vi "11_LAYOUT_COVID_19_BOTÓN.vi"() -> ()   [LabVIEW 2019]
panel:
  in  "vi path":path
  out "Numeric":i32
  in  "INT_TAB":bool
  in  "Tab Control":enum32{"Page 1", "Page 2"}(tab)
  out "Boolean":bool
  out "Boolean 2":bool
  in  "stop":bool
  # "LAYOUT --> TAB/SUB"
  # "SELECTOR TAB"
  # "(C) 2020"
  # "J.LUIS PÉREZ DEL VAL"
  # "GIF ANIMADO"
  # "KIT o CALENDARIO?..."
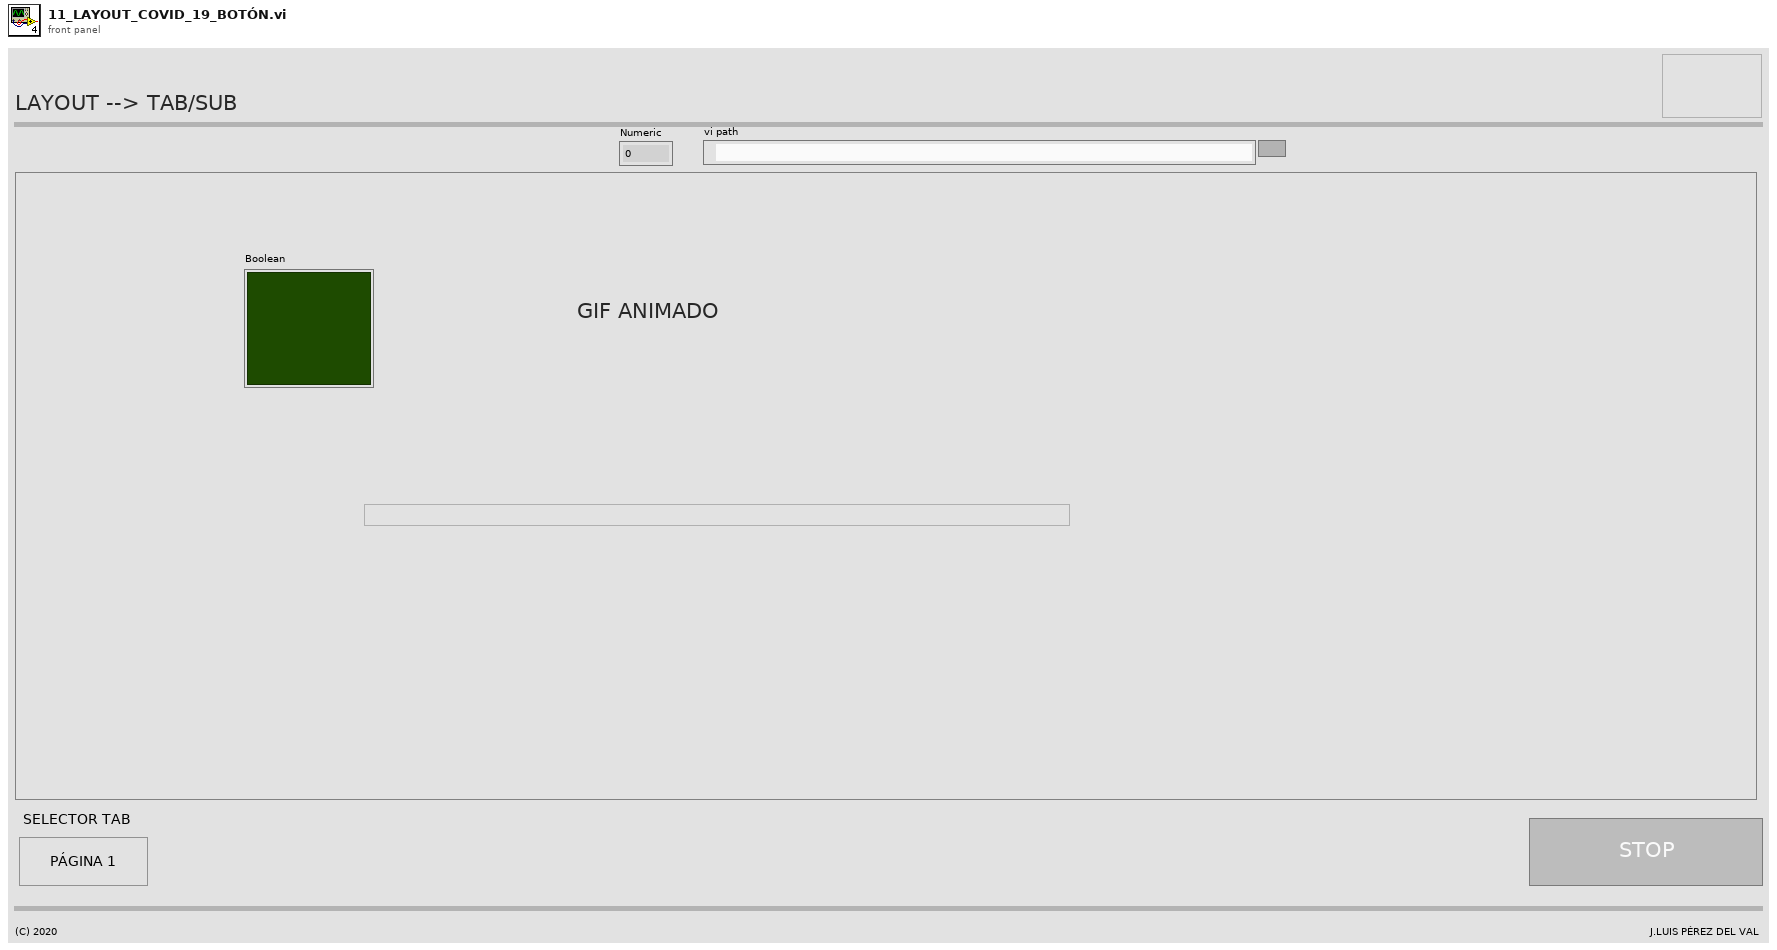
[diagram p1: front panel]
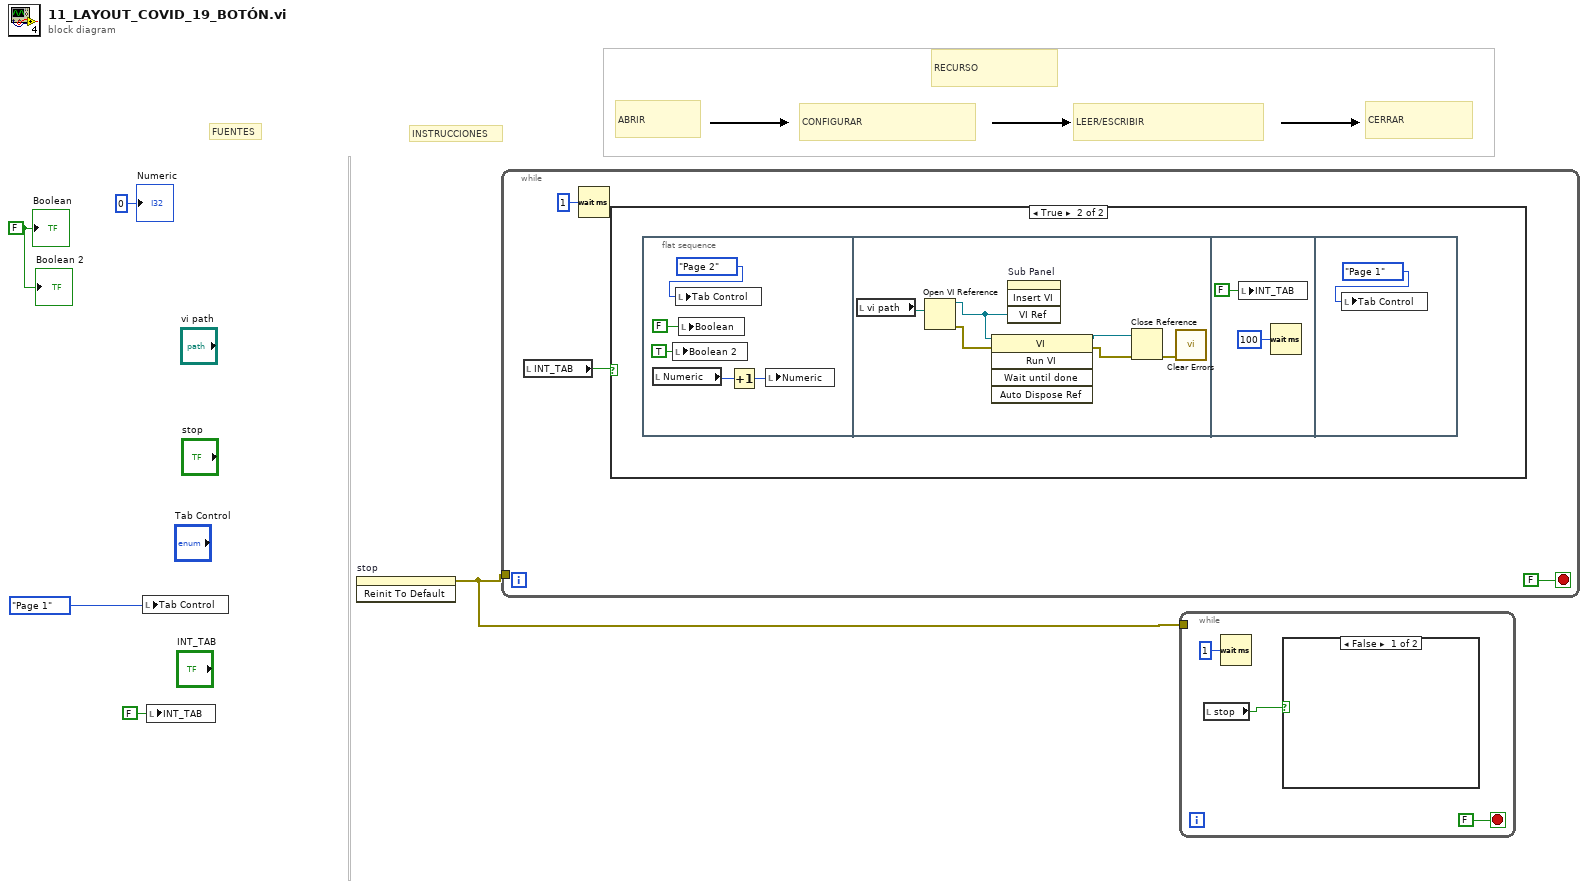
[diagram p0: block diagram]
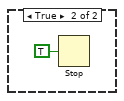
[diagram p2: hidden frame]
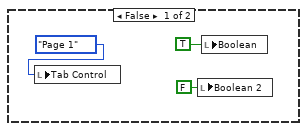
[diagram p3: hidden frame]
diagram:
  w2 = FALSE ("Boolean")
  # "RECURSO"
  # "CERRAR"
  # "LEER/ESCRIBIR"
  # "CONFIGURAR"
  # "ABRIR"
  # "INSTRUCCIONES"
  # "FUENTES"
  n1 = local write "Tab Control"(enum32{"Page 1", "Page 2"}."Page 1" ("Tab Control 2")) -> ()
  n2 = local write "INT_TAB"(FALSE ("INT_TAB")) -> ()
  n3 = invoke on="stop" class="Bool (strict)" method="Reinit To Default"() -> (error out=w5:errorcluster)  [unwired: 3 in, 2 out]
  n4 = while {
    tunnel: w5 -> [_]
    stop <- FALSE stop-if-true
    n5 = local read "INT_TAB"() -> (w6:bool)
    n6 = Wait (ms)(milliseconds to wait=u32 1) -> ()  [unwired: 1 out]
    n7 = case shown="True" w6 {
      frame False {
        n8 = local write "Tab Control"(enum32{"Page 1", "Page 2"}."Page 1" ("Tab Control 2")) -> ()
        n9 = local write "Boolean 2"(FALSE ("INT_TAB")) -> ()
        n10 = local write "Boolean"(TRUE ("INT_TAB")) -> ()
      }
      frame True {
        n11 = flat-sequence {
          frame #0 {
            n12 = local read "Numeric"() -> (w14:i32)
            n13 = local write "Boolean 2"(TRUE ("INT_TAB")) -> ()
            n14 = local write "Tab Control"(enum32{"Page 1", "Page 2"}."Page 2" ("Tab Control 2")) -> ()
            n15 = local write "Boolean"(FALSE ("INT_TAB")) -> ()
            n16 = Increment(x=w14) -> (x+1=w13:i32)
            n17 = local write "Numeric"(w13) -> ()
          }
          frame #1 {
            n18 = local read "vi path"() -> (w20:path)
            n19 = Open VI Reference(vi path=w20) -> (vi reference=w19:refnum<vi>, error out=w18:errorcluster)  [unwired: 5 in]
            n20 = invoke class="VI" method="Run VI"(reference=w19, error in=w18) -> (reference out=w21:refnum<vi>, error out=w22:errorcluster)  [unwired: 3 in, 3 out]
            n21 = invoke on="Sub Panel" class="SubPnl" method="Insert VI"("VI Ref"=w19) -> ()  [unwired: 3 in, 4 out]
            n22 = Close Reference(reference=w21, error in (no error)=w22) -> (error out=w17:errorcluster)
            n23 = call <vilib>:"Clear Errors.vi"("error in (no error)"=w17) -> ()  [unwired: 5 in, 2 out]
          }
          frame #2 {
            n24 = local write "INT_TAB"(FALSE ("INT_TAB")) -> ()
            n25 = Wait (ms)(milliseconds to wait=u32 100) -> ()  [unwired: 1 out]
          }
          frame #3 {
            n26 = local write "Tab Control"(enum32{"Page 1", "Page 2"}."Page 1" ("Tab Control 2")) -> ()
          }
        }
      }
    }
  }
  n27 = while {
    tunnel: w5 -> [_]
    stop <- FALSE stop-if-true
    n28 = local read "stop"() -> (w26:bool)
    n29 = Wait (ms)(milliseconds to wait=u32 1) -> ()  [unwired: 1 out]
    n30 = case shown="False" w26 {
      frame False {
      }
      frame True {
        n31 = Stop(stop? (T)=TRUE) -> ()
      }
    }
  }
  "Boolean" <- w2
  "Boolean 2" <- w2
  "Numeric" <- 0 ("Numeric")
